vi "GetBlock.vi"(7 "Position":cluster{"X":dbl, "Y":dbl, "Theta":dbl}, 8 "Error/Flow Out":errorcluster, 9 "Theta":dbl, 10 "Change":bool, 11 "Right Arm":bool) -> (0 "Error/Flow Out 2":errorcluster, 2 "New Position":cluster{"X":dbl, "Y":dbl, "Theta":dbl})   [LabVIEW 2018]
uses:
  2353369a-33d7-4dbc-85ab-8d997f1fe143.vi
  <vilib>/Analysis/NI_AALPro.lvlib
  <vilib>/Analysis/coordinate.llb/2D Cartesian Coordinate Shift (Scalar).vi
  <vilib>/Analysis/coordinate.llb/2D Cartesian Coordinate Rotation (Scalar).vi
  <vilib>/vision/NI_Vision_Development_Module.lvlib
  <vilib>/vision/driver/NI_Vision_Acquisition_Software.lvlib
  <resource>/objmgr/imaqdx.rc
panel:
  out "element":string
  out "Image":T1(plugin-control)
  out "Camera Data":dbl[][](array[numeric]) format="%.2f"
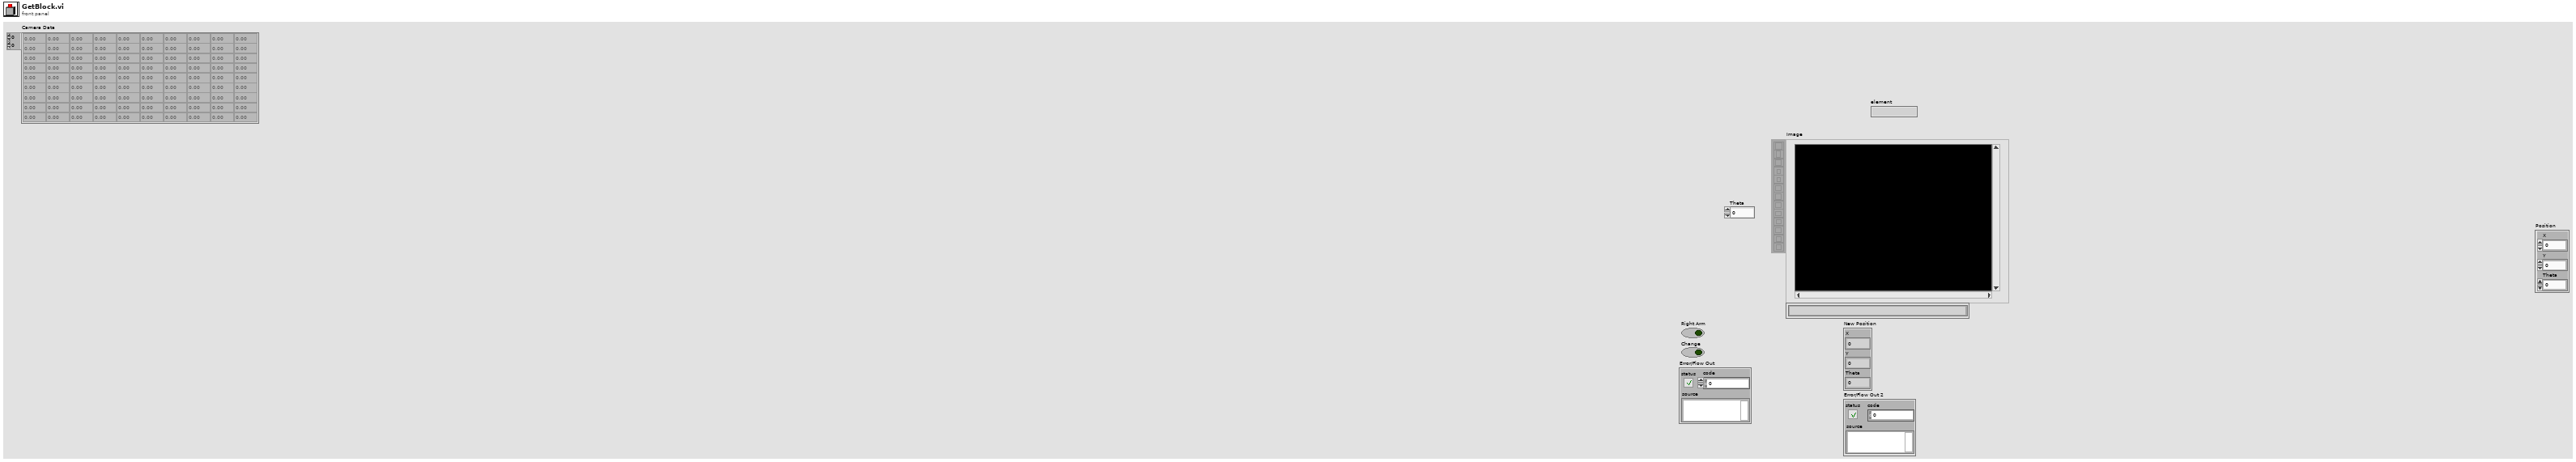
[diagram p1: front panel]
types:
  T1 = typedef "IMAQ Image.ctl" = refnum<image>
  T2 = typedef "IMAQdx.ctl" = refnum<k21>
  T3 = typedef "Particle Parameters" = i32
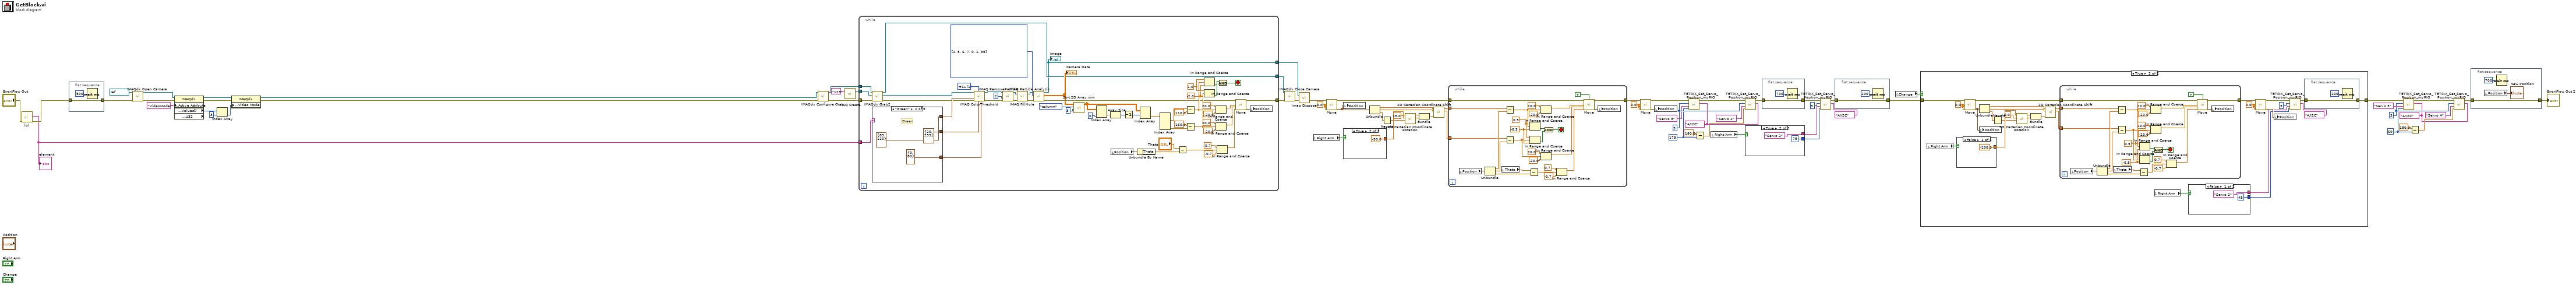
[diagram p0: block diagram]
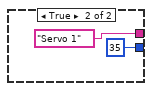
[diagram p3: hidden frame]
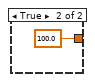
[diagram p4: hidden frame]
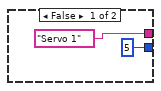
[diagram p5: hidden frame]
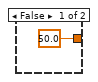
[diagram p6: hidden frame]
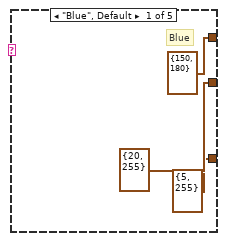
[diagram p7: hidden frame]
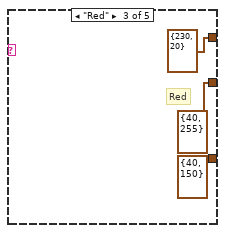
[diagram p8: hidden frame]
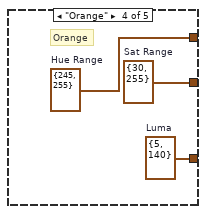
[diagram p9: hidden frame]
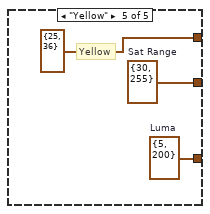
[diagram p10: hidden frame]
diagram:
  w33 = u8 60 ("Servo 4 Position (0 - 180 degrees)")
  w31 = u8 3 ("Controller ID#  (I2C Address)")
  w30 = tag "A/I2C" ("myRIO MXP Port A/B")
  w46 = 0.0 ("x (mm/s)")
  w57 = u8 175 ("Servo 4 Position (0 - 180 degrees)")
  w60 = u8 3 ("Controller ID#  (I2C Address)")
  w61 = tag "A/I2C" ("myRIO MXP Port A/B")
  w72 = 0.0 ("x (mm/s)")
  n1 = call "lol.vi"("error in"="Error/Flow Out") -> ("error out"=w4:errorcluster, "element"=w3:string)  [unwired: 9 in]
  "element" <- w3
  n2 = flat-sequence {
    tunnel: [w73] -> w8
    tunnel: w4 -> [w73]
    frame #0 {
      n3 = Wait (ms)(milliseconds to wait=u32 500) -> ()  [unwired: 1 out]
    }
  }
  n4 = call <vilib>:"IMAQdx Open Camera.vi"("error in"=w8, "Session In"=refnum<k21> "cam1" ("Camera Name")) -> ("error out"=w24:errorcluster, "Session Out"=w22:T2)  [unwired: 1 in, 7 out]
  n5 = property class="IMAQdx" props=["Camera Attributes:Active Attribute", "Camera Attributes:Enum:Values[]", "Camera Attributes:Value:U32"](reference=w22, error in=w24, "Camera Attributes:Active Attribute"="VideoMode" ("ActiveAttribute")) -> (reference out=w19:T2, error out=w18:errorcluster, "Camera Attributes:Enum:Values[]"=w15:u32[])  [unwired: 1 out]
  n6 = Index Array(array=w15, index=3 ("Video Modes")) -> (element=w16:u32)
  n7 = property class="IMAQdx"(reference=w19, error in=w18, "Acquisition Attributes:Video Mode"=w16) -> (reference out=w2:T2, error out=w1:errorcluster)
  n8 = call <vilib>:"IMAQdx Configure Grab.vi"("error in"=w1, "Session In"=w2) -> ("error out"=w7:errorcluster, "Session Out"=w6:T2)  [unwired: 8 in]
  n9 = call "IMAQ Create"("Image Name"="123") -> ("New Image"=w11:T1)  [unwired: 3 in, 2 out]
  n10 = while {
    tunnel: [w106] -> w13
    tunnel: w11 -> [w80]
    tunnel: [w79] -> w10
    tunnel: [w76] -> w9
    tunnel: w7 -> [w78]
    tunnel: w6 -> [w77]
    tunnel: w3 -> [w75]
    stop <- w83 stop-if-true
    w87 = T3[] [4, 5, 6, 7, 0, 1, 35] items=["Center of Mass X", "Center of Mass Y", "First Pixel X", "First Pixel Y", "Bounding Rect Left", "Bounding Rect Top", "Bounding Rect Right", "Bounding Rect Bottom", "Max Feret Diameter Start X", "Max Feret Diameter Start Y", "Max Feret Diameter End X", "Max Feret Diameter End Y", "Max Horiz. Segment Length Left", "Max Horiz. Segment Length Right", "Max Horiz. Segment Length Row", "-", "Bounding Rect Width", "Bounding Rect Height", "Bounding Rect Diagonal", "Perimeter", "Convex Hull Perimeter", "Holes' Perimeter", "Max Feret Diameter", "Equivalent Ellipse Major Axis", "Equivalent Ellipse Minor Axis", "Equivalent Ellipse Minor Axis (Feret)", "Equivalent Rect Long Side", "Equivalent Rect Short Side", "Equivalent Rect Diagonal", "Equivalent Rect Short Side (Feret)", "Average Horiz. Segment Length", "Average Vert. Segment Length", "Hydraulic Radius", "Waddel Disk Diameter", "-", "Area", "Holes' Area", "Particle & Holes' Area", "Convex Hull Area", "Image Area", "-", "Number of Holes", "Number of Horiz. Segments", "Number of Vert. Segments", "-", "Orientation", "Max Feret Diameter Orientation", "-", "% Area/Image Area", "% Area/(Particle & Holes' Area)", "Ratio of Equivalent Ellipse Axes", "Ratio of Equivalent Rect Sides", "-", "Elongation Factor", "Compactness Factor", "Heywood Circularity Factor", "Type Factor", "-", "Sum X", "Sum Y", "Sum XX", "Sum XY", "Sum YY", "Sum XXX", "Sum XXY", "Sum XYY", "Sum YYY", "-", "Moment of Inertia XX", "Moment of Inertia XY", "Moment of Inertia YY", "Moment of Inertia XXX", "Moment of Inertia XXY", "Moment of Inertia XYY", "Moment of Inertia YYY", "Norm. Moment of Inertia XX", "Norm. Moment of Inertia XY", "Norm. Moment of Inertia YY", "Norm. Moment of Inertia XXX", "Norm. Moment of Inertia XXY", "Norm. Moment of Inertia XYY", "Norm. Moment of Inertia YYY", "Hu Moment 1", "Hu Moment 2", "Hu Moment 3", "Hu Moment 4", "Hu Moment 5", "Hu Moment 6", "Hu Moment 7"] ("Pixel Measurements")
    w97 = u16 1 items=["RGB", "HSL", "HSV", "HSI"] ("Color Mode")
    w110 = -2.0 ("lower limit")
    w111 = 2.0 ("upper limit")
    n11 = call <vilib>:"IMAQdx Grab2.vi"("error in"=w78, "Image In"=w80, "Session In"=w77) -> ("error out"=w81:errorcluster, "Image Out"=w82:T1, "Session Out"=w79:T2)  [unwired: 5 in, 1 out]
    n12 = case shown="\"Green\"" w75 {
      tunnel: [cluster{"Lower value":i32, "Upper value":i32} {"Lower value"=150, "Upper value"=180} ("Hue Range") cluster{"Lower value":i32, "Upper value":i32} {"Lower value"=83, "Upper value"=110} ("Hue Range") cluster{"Lower value":i32, "Upper value":i32} {"Lower value"=230, "Upper value"=20} ("Hue Range") w142 cluster{"Lower value":i32, "Upper value":i32} {"Lower value"=25, "Upper value"=36} ("Hue Range")] -> w96
      tunnel: [cluster{"Lower value":i32, "Upper value":i32} {"Lower value"=20, "Upper value"=255} ("Sat Range") cluster{"Lower value":i32, "Upper value":i32} {"Lower value"=20, "Upper value"=255} ("Sat Range") cluster{"Lower value":i32, "Upper value":i32} {"Lower value"=40, "Upper value"=255} ("Sat Range") w141 w144] -> w95
      tunnel: [cluster{"Lower value":i32, "Upper value":i32} {"Lower value"=5, "Upper value"=255} ("Luma") cluster{"Lower value":i32, "Upper value":i32} {"Lower value"=0, "Upper value"=80} ("Luma") cluster{"Lower value":i32, "Upper value":i32} {"Lower value"=40, "Upper value"=150} ("Luma") w140 w143] -> w94
      frame "Blue", Default {
        # "Blue"
      }
      frame "Green" {
        # "Green"
      }
      frame "Red" {
        # "Red"
      }
      frame "Orange" {
        w140 = cluster{"Lower value":i32, "Upper value":i32} {"Lower value"=5, "Upper value"=140}  # Luma
        w141 = cluster{"Lower value":i32, "Upper value":i32} {"Lower value"=30, "Upper value"=255}  # Sat Range
        w142 = cluster{"Lower value":i32, "Upper value":i32} {"Lower value"=245, "Upper value"=255}  # Hue Range
        # "Orange"
      }
      frame "Yellow" {
        w143 = cluster{"Lower value":i32, "Upper value":i32} {"Lower value"=5, "Upper value"=200}  # Luma
        w144 = cluster{"Lower value":i32, "Upper value":i32} {"Lower value"=30, "Upper value"=255}  # Sat Range
        # "Yellow"
      }
    }
    n13 = call "IMAQ ColorThreshold"("Blue or Luma or Val or Inten Range"=w94, "Green or Sat Range"=w95, "Color Mode"=w97, "error in (no error)"=w81, "Red or Hue Range"=w96, "Image Src"=w82) -> ("error out"=w93:errorcluster, "Image Dst Out"=w92:T1)  [unwired: 4 in]
    n14 = call "IMAQ RemoveParticle"("error in (no error)"=w93, "Number of Erosion"=2, "Image Src"=w92) -> ("error out"=w91:errorcluster, "Image Dst Out"=w90:T1)  [unwired: 7 in]
    n15 = call "IMAQ FillHole"("error in (no error)"=w91, "Image Src"=w90) -> ("error out"=w89:errorcluster, "Image Dst Out"=w88:T1)  [unwired: 4 in]
    n16 = call "IMAQ Particle Analysis"("error in (no error)"=w89, "Pixel Measurements"=w87, "Image"=w88) -> ("error out"=w85:errorcluster, "Particle Measurements (Pixels)"=w84:dbl[][], "Image Out (duplicate)"=w76:T1)  [unwired: 3 in, 3 out]
    "Camera Data" <- w84
    "Image" <- w76
    n17 = call "Sort 2D Array.vim"("index"=3, "dimension to index (column)"=enum16{"column", "row"}."column", "2D array"=w84) -> ("sorted 2D array"=w128:dbl[][])  [unwired: 7 in, 1 out]
    n18 = Index Array(array=w128, index (col)=0 ("disabled index (col)")) -> (element=w126:dbl[])  [unwired: 1 in]
    n19 = Array Size(array=w126) -> (size(s)=w125:i32)
    n20 = local read "Position"() -> (w118:cluster{"X":dbl, "Y":dbl, "Theta":dbl})
    n21 = Decrement(x=w125) -> (x-1=w124:i32)
    n22 = Unbundle By Name(w118) -> ("Theta"=w117:dbl)
    n23 = Index Array(array=w128, index (row)=w124) -> (element=w123:dbl[])  [unwired: 1 in]
    n24 = Index Array(array=w123) -> (element #1=w102:dbl, element #4=w99:dbl)  [unwired: 4 in, 2 out]
    n25 = Subtract(x="Theta", y=w117) -> (x-y=w116:dbl)
    n26 = Subtract(x=w102, y=110.0 ("x")) -> (x-y=w109:dbl)
    n27 = Subtract(x=160.0 ("y"), y=w99) -> (x-y=w112:dbl)
    n28 = In Range and Coerce(upper limit=w111, x=w109, lower limit=w110) -> (In Range?=w107:bool)  [unwired: 1 out]
    n29 = In Range and Coerce(upper limit=w111, x=w112, lower limit=w110) -> (In Range?=w108:bool)  [unwired: 1 out]
    n30 = In Range and Coerce(upper limit=20.0, x=w109, lower limit=-20.0) -> (coerced(x)=w103:dbl)  [unwired: 1 out]
    n31 = In Range and Coerce(upper limit=20.0, x=w112, lower limit=-20.0) -> (coerced(x)=w104:dbl)  [unwired: 1 out]
    n32 = In Range and Coerce(upper limit=0.7, x=w116, lower limit=-0.7) -> (coerced(x)=w113:dbl)  [unwired: 1 out]
    n33 = And(x=w108, y=w107) -> (x .and. y?=w83:bool)
    n34 = call "Move.vi"("Error/Flow In"=w85, "x (mm/s)"=w103, "y (mm/s)"=w104, "theta (rad/s)"=w113) -> ("Error/Flow Out"=w106:errorcluster, "Position"=w105:cluster{"X":dbl, "Y":dbl, "Theta":dbl})  [unwired: 10 in]
    n35 = local write "Position"(w105) -> ()
  }
  n36 = call <vilib>:"IMAQdx Close Camera.vi"("error in"=w13, "Session In"=w10) -> ("error out"=w14:errorcluster)  [unwired: 9 out]
  n37 = call "Imaq Dispose"("Image"=w9, "error in (no error)"=w14) -> ("error out"=w12:errorcluster)  [unwired: 4 in]
  n38 = local read "Right Arm"() -> (w52:bool)
  n39 = call "Move.vi"("Error/Flow In"=w12, "x (mm/s)"=w72, "y (mm/s)"=w72, "theta (rad/s)"=w72) -> ("Error/Flow Out"=w62:errorcluster, "Position"=w71:cluster{"X":dbl, "Y":dbl, "Theta":dbl})  [unwired: 10 in]
  n40 = local write "Position"(w71) -> ()
  n41 = case shown="True" w52 {
    tunnel: [50.0 -50.0] -> w51
    frame False {
    }
    frame True {
    }
  }
  n42 = Unbundle(w71) -> ("X"=w66:dbl, "Y"=w65:dbl, "Theta"=w25:dbl)
  n43 = Negate(x=w25) -> (-x=w26:dbl)
  n44 = call-poly <vilib>:"2D Cartesian Coordinate Rotation.vi"("theta"=w26, "y"=15.0, "x"=w51) -> ("y out"=w68:dbl, "x out"=w69:dbl)  [unwired: 6 in, 1 out]
  n45 = Bundle("x out"=w69, "y out"=w68) -> (w67:cluster{"x out":dbl, "y out":dbl})  [unwired: 1 in]
  n46 = call-poly <vilib>:"2D Cartesian Coordinate Shift.vi"("shift"=w67, "y"=w65, "x"=w66) -> ("y out"=w63:dbl, "x out"=w64:dbl)  [unwired: 6 in, 1 out]
  n47 = while {
    tunnel: w64 -> [w173]
    tunnel: w63 -> [w167]
    tunnel: w62 -> [w154]
    tunnel: [w151] -> w49
    stop <- w162 stop-if-true
    w149 = -0.5 ("upper limit")
    w150 = 0.5 ("upper limit")
    n48 = local read "Position"() -> (w175:cluster{"X":dbl, "Y":dbl, "Theta":dbl})
    n49 = Unbundle(w175) -> ("X"=w174:dbl, "Y"=w168:dbl, "Theta"=w166:dbl)
    n50 = local read "Theta"() -> (w148:dbl)
    n51 = Subtract(x=w173, y=w174) -> (x-y=w158:dbl)
    n52 = Subtract(x=w167, y=w168) -> (x-y=w159:dbl)
    n53 = Subtract(x=w148, y=w166) -> (x-y=w165:dbl)
    n54 = In Range and Coerce(upper limit=w150, x=w158, lower limit=w149) -> (In Range?=w160:bool)  [unwired: 1 out]
    n55 = In Range and Coerce(upper limit=w150, x=w159, lower limit=w149) -> (In Range?=w161:bool)  [unwired: 1 out]
    n56 = In Range and Coerce(upper limit=20.0, x=w158, lower limit=-20.0) -> (coerced(x)=w155:dbl)  [unwired: 1 out]
    n57 = In Range and Coerce(upper limit=20.0, x=w159, lower limit=-20.0) -> (coerced(x)=w156:dbl)  [unwired: 1 out]
    n58 = And(x=w160, y=w161) -> (x .and. y?=w162:bool)
    n59 = In Range and Coerce(upper limit=0.7, x=w165, lower limit=-0.7 ("upper limit")) -> (coerced(x)=w157:dbl)  [unwired: 1 out]
    n60 = call "Move.vi"("Error/Flow In"=w154, "Relative to Global Frame"=TRUE, "x (mm/s)"=w155, "y (mm/s)"=w156, "theta (rad/s)"=w157) -> ("Error/Flow Out"=w151:errorcluster, "Position"=w153:cluster{"X":dbl, "Y":dbl, "Theta":dbl})  [unwired: 9 in]
    n61 = local write "Position"(w153) -> ()
  }
  n62 = call "Move.vi"("Error/Flow In"=w49, "x (mm/s)"=w46, "y (mm/s)"=w46, "theta (rad/s)"=w46) -> ("Error/Flow Out"=w48:errorcluster, "Position"=w47:cluster{"X":dbl, "Y":dbl, "Theta":dbl})  [unwired: 10 in]
  n63 = local write "Position"(w47) -> ()
  n64 = call <vilib>:"TETRIX_Set_Servo_Position_myRIO.vi"("myRIO MXP Port A/B"=w61, "Set Servo Position (0 - 180 degrees)"=w57, "Select Channel"="Servo 3", "Controller ID#  (I2C Address)"=w60, "Error/Flow In"=w48) -> ("Error/Flow Out"=w53:errorcluster)  [unwired: 2 in]
  n65 = Subtract(x=180.0, y=w57) -> (x-y=w58:dbl)
  n66 = local read "Right Arm"() -> (w50:bool)
  n67 = call <vilib>:"TETRIX_Set_Servo_Position_myRIO.vi"("myRIO MXP Port A/B"=w61, "Set Servo Position (0 - 180 degrees)"=w58, "Select Channel"="Servo 4", "Controller ID#  (I2C Address)"=w60, "Error/Flow In"=w53) -> ("Error/Flow Out"=w59:errorcluster)  [unwired: 2 in]
  n68 = case shown="True" w50 {
    tunnel: ["Servo 1" ("Select Channel") "Servo 2" ("Select Channel")] -> w45
    tunnel: [u8 5 ("Set Servo Position (0 - 180 degrees)") u8 75 ("Set Servo Position (0 - 180 degrees)")] -> w44
    frame False {
    }
    frame True {
    }
  }
  n69 = flat-sequence {
    tunnel: w59 -> [w180]
    tunnel: [w180] -> w43
    frame #0 {
      n70 = Wait (ms)(milliseconds to wait=u32 700) -> ()  [unwired: 1 out]
    }
  }
  n71 = call <vilib>:"TETRIX_Set_Servo_Position_myRIO.vi"("myRIO MXP Port A/B"=tag "A/I2C", "Set Servo Position (0 - 180 degrees)"=w44, "Select Channel"=w45, "Controller ID#  (I2C Address)"=u8 3, "Error/Flow In"=w43) -> ("Error/Flow Out"=w40:errorcluster)  [unwired: 2 in]
  n72 = flat-sequence {
    tunnel: w40 -> [w182]
    tunnel: [w182] -> w39
    frame #0 {
      n73 = Wait (ms)(milliseconds to wait=u32 200) -> ()  [unwired: 1 out]
    }
  }
  n74 = local read "Change"() -> (w38:bool)
  n75 = case shown="True" w38 {
    tunnel: w39 -> [w184 w195]
    tunnel: [w184 w187] -> w29
    frame False {
    }
    frame True {
      w211 = 0.0 ("x (mm/s)")
      w196 = 0.0 ("x (mm/s)")
      n76 = local read "Right Arm"() -> (w207:bool)
      n77 = case shown="False" w207 {
        tunnel: [-100.0 100.0] -> w208
        frame False {
        }
        frame True {
        }
      }
      n78 = call "Move.vi"("Error/Flow In"=w195, "x (mm/s)"=w196, "y (mm/s)"=w196, "theta (rad/s)"=w196) -> ("Error/Flow Out"=w206:errorcluster, "Position"=w197:cluster{"X":dbl, "Y":dbl, "Theta":dbl})  [unwired: 10 in]
      n79 = Unbundle(w197) -> ("X"=w202:dbl, "Y"=w203:dbl, "Theta"=w185:dbl)
      n80 = local write "Position"(w197) -> ()
      n81 = Negate(x=w185) -> (-x=w186:dbl)
      n82 = call-poly <vilib>:"2D Cartesian Coordinate Rotation.vi"("theta"=w186, "y"=0.0, "x"=w208) -> ("y out"=w200:dbl, "x out"=w199:dbl)  [unwired: 6 in, 1 out]
      n83 = Bundle("x out"=w199, "y out"=w200) -> (w201:cluster{"x out":dbl, "y out":dbl})  [unwired: 1 in]
      n84 = call-poly <vilib>:"2D Cartesian Coordinate Shift.vi"("shift"=w201, "y"=w203, "x"=w202) -> ("y out"=w205:dbl, "x out"=w204:dbl)  [unwired: 6 in, 1 out]
      n85 = while {
        tunnel: w204 -> [w245]
        tunnel: w205 -> [w239]
        tunnel: w206 -> [w226]
        tunnel: [w223] -> w209
        stop <- w234 stop-if-true
        w221 = -0.5 ("upper limit")
        w222 = 0.5 ("upper limit")
        n86 = local read "Position"() -> (w247:cluster{"X":dbl, "Y":dbl, "Theta":dbl})
        n87 = Unbundle(w247) -> ("X"=w246:dbl, "Y"=w240:dbl, "Theta"=w238:dbl)
        n88 = local read "Theta"() -> (w220:dbl)
        n89 = Subtract(x=w245, y=w246) -> (x-y=w230:dbl)
        n90 = Subtract(x=w239, y=w240) -> (x-y=w231:dbl)
        n91 = Subtract(x=w220, y=w238) -> (x-y=w237:dbl)
        n92 = In Range and Coerce(upper limit=w222, x=w230, lower limit=w221) -> (In Range?=w232:bool)  [unwired: 1 out]
        n93 = In Range and Coerce(upper limit=w222, x=w231, lower limit=w221) -> (In Range?=w233:bool)  [unwired: 1 out]
        n94 = In Range and Coerce(upper limit=20.0, x=w230, lower limit=-20.0) -> (coerced(x)=w227:dbl)  [unwired: 1 out]
        n95 = In Range and Coerce(upper limit=20.0, x=w231, lower limit=-20.0) -> (coerced(x)=w228:dbl)  [unwired: 1 out]
        n96 = And(x=w232, y=w233) -> (x .and. y?=w234:bool)
        n97 = In Range and Coerce(upper limit=0.7, x=w237, lower limit=-0.7 ("upper limit")) -> (coerced(x)=w229:dbl)  [unwired: 1 out]
        n98 = call "Move.vi"("Error/Flow In"=w226, "Relative to Global Frame"=TRUE, "x (mm/s)"=w227, "y (mm/s)"=w228, "theta (rad/s)"=w229) -> ("Error/Flow Out"=w223:errorcluster, "Position"=w225:cluster{"X":dbl, "Y":dbl, "Theta":dbl})  [unwired: 9 in]
        n99 = local write "Position"(w225) -> ()
      }
      n100 = local read "Right Arm"() -> (w189:bool)
      n101 = case shown="False" w189 {
        tunnel: ["Servo 2" ("Select Channel") "Servo 1" ("Select Channel")] -> w190
        tunnel: [u8 45 ("Set Servo Position (0 - 180 degrees)") u8 35 ("Set Servo Position (0 - 180 degrees)")] -> w191
        frame False {
        }
        frame True {
        }
      }
      n102 = call "Move.vi"("Error/Flow In"=w209, "x (mm/s)"=w211, "y (mm/s)"=w211, "theta (rad/s)"=w211) -> ("Error/Flow Out"=w188:errorcluster, "Position"=w210:cluster{"X":dbl, "Y":dbl, "Theta":dbl})  [unwired: 10 in]
      n103 = local write "Position"(w210) -> ()
      n104 = call <vilib>:"TETRIX_Set_Servo_Position_myRIO.vi"("myRIO MXP Port A/B"=tag "A/I2C", "Set Servo Position (0 - 180 degrees)"=w191, "Select Channel"=w190, "Controller ID#  (I2C Address)"=u8 3, "Error/Flow In"=w188) -> ("Error/Flow Out"=w194:errorcluster)  [unwired: 2 in]
      n105 = flat-sequence {
        tunnel: w194 -> [w212]
        tunnel: [w212] -> w187
        frame #0 {
          n106 = Wait (ms)(milliseconds to wait=u32 200) -> ()  [unwired: 1 out]
        }
      }
    }
  }
  n107 = call <vilib>:"TETRIX_Set_Servo_Position_myRIO.vi"("myRIO MXP Port A/B"=w30, "Set Servo Position (0 - 180 degrees)"=w33, "Select Channel"="Servo 3", "Controller ID#  (I2C Address)"=w31, "Error/Flow In"=w29) -> ("Error/Flow Out"=w37:errorcluster)  [unwired: 2 in]
  n108 = Subtract(x=180.0, y=w33) -> (x-y=w32:dbl)
  n109 = call <vilib>:"TETRIX_Set_Servo_Position_myRIO.vi"("myRIO MXP Port A/B"=w30, "Set Servo Position (0 - 180 degrees)"=w32, "Select Channel"="Servo 4", "Controller ID#  (I2C Address)"=w31, "Error/Flow In"=w37) -> ("Error/Flow Out"=w28:errorcluster)  [unwired: 2 in]
  n110 = flat-sequence {
    tunnel: w28 -> [w249]
    tunnel: [w249] -> w27
    frame #0 {
      n111 = local read "Position"() -> (→"New Position":cluster{"X":dbl, "Y":dbl, "Theta":dbl})
      n112 = Wait (ms)(milliseconds to wait=u32 700) -> ()  [unwired: 1 out]
    }
  }
  "Error/Flow Out 2" <- w27
